vi "SetSave.vi"(8 "error in (no error)":errorcluster, 10 "on/off":T1, 11 "Photometrics Cam v2 in":refnum<class "Photometrics_CH-250_Cam.lvclass">) -> (0 "error out":errorcluster, 2 "on/off (out)":T1, 3 "Photometrics Cam v2 out":refnum<class "Photometrics_CH-250_Cam.lvclass">)   [LabVIEW 2013, in "Photometrics_CH-250_Cam.lvclass"]
uses:
  Photometrics_CH-250_Cam.lvclass
  shared/OnOffTypeDef.ctl
  Photometrics_CH-250_Cam.lvclass/Photometrics_CH-250_Cam.ctl
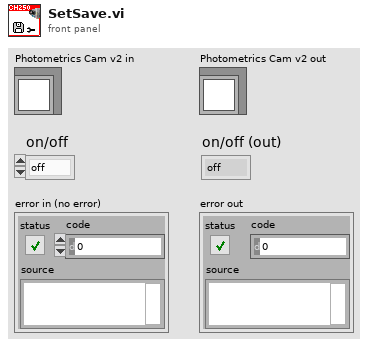
[diagram p1: front panel]
types:
  T1 = typedef "OnOffTypeDef.ctl" = enum16{"off", "on"}
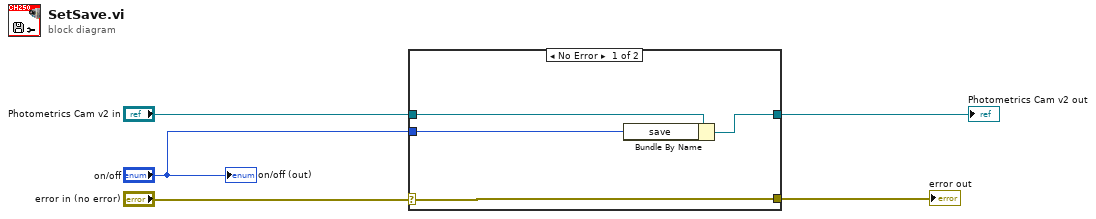
[diagram p0: block diagram]
diagram:
  n1 = case shown="No Error" "error in (no error)" {
    selector: "error in (no error)" -> [w6 w11]
    tunnel: [w9 w10] -> w2
    tunnel: "Photometrics Cam v2 in" -> [w8 w10]
    tunnel: "on/off" -> [w7 _]
    tunnel: [w6 w11] -> w5
    frame No Error {
      n2 = Bundle By Name(cluster=w8, "save"=w7) -> (w9:refnum<class "Photometrics_CH-250_Cam.lvclass">)
    }
    frame Error {
    }
  }
  "error out" <- w5
  "Photometrics Cam v2 out" <- w2
  "on/off (out)" <- "on/off"
